vi "Unique.vi"   [LabVIEW 2009]
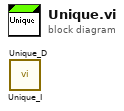
[diagram p0: block diagram]
diagram:
  n1 = call "Unique_I.vi"() -> ()  [unwired: 11 in, 1 out]
  n2 = call "Unique_D.vi"() -> ()  [unwired: 11 in, 1 out]
